vi "Start AsyncSum.vi"(7 "Opeation":string, 8 "error in (no error)":errorcluster, 9 "B":i32, 10 "A":i32, 11 "Skeleton in":refnum<class "Skeleton.lvclass">) -> (0 "error out":errorcluster, 2 "AsyncSum Event Register":refnum<event-registration>, 3 "Skeleton out":refnum<class "Skeleton.lvclass">)   [LabVIEW 2016, in "Skeleton.lvlib" / "Skeleton.lvclass"]
uses:
  Skeleton.lvclass
  Skeleton.lvclass/Skeleton.ctl
  Active Thread Configuration.ctl
  DemoSkeleton/DemoSkeleton.lvlib
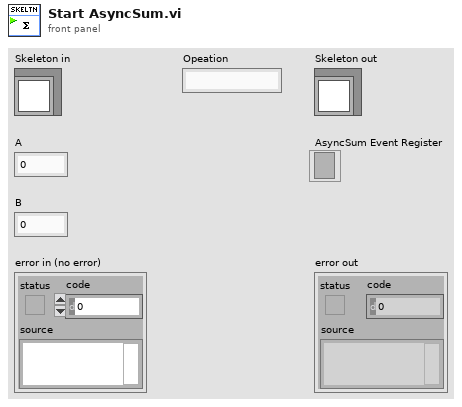
[diagram p1: front panel]
types:
  T1 = typedef "Skeleton.lvlib/Skeleton.lvclass/Active Thread Configuration.ctl" = cluster{"Operation":string, "Handle":u64, "LVUserEvent CallBack Reference":refnum<user-event>}
  T2 = typedef "Skeleton.lvlib/Skeleton.lvclass/Private Data.ctl" = cluster{"DLL path":path, "Active Thread Map":variant}
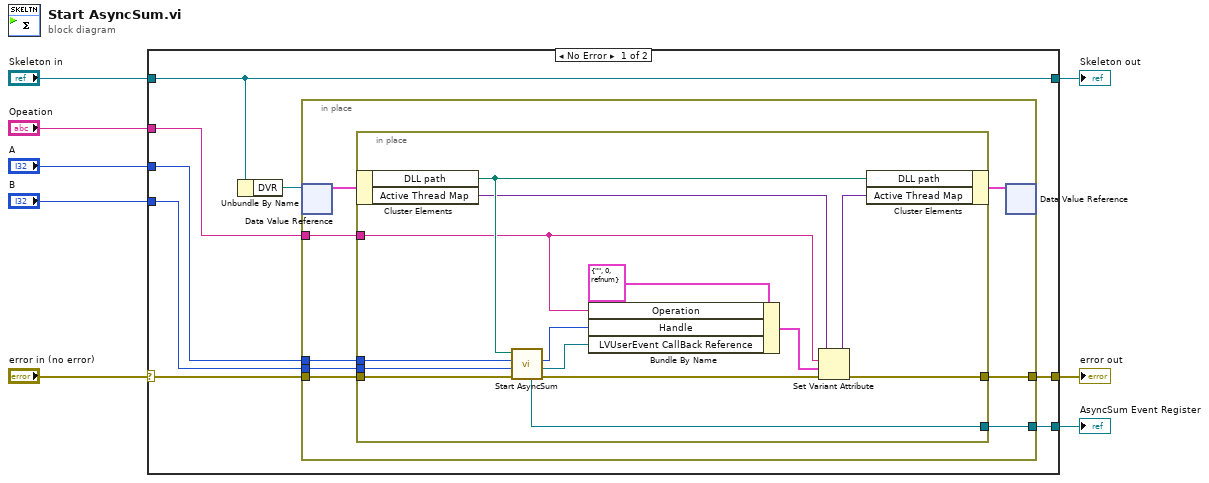
[diagram p0: block diagram]
diagram:
  n1 = case shown="No Error" "error in (no error)" {
    selector: "error in (no error)" -> [w16 w40]
    tunnel: [w15 w40] -> w8
    tunnel: [w12 w39] -> w7
    tunnel: "Skeleton in" -> [w12 w39]
    tunnel: "A" -> [w13 _]
    tunnel: "B" -> [w14 _]
    tunnel: "Opeation" -> [w10 _]
    tunnel: [w9 _] -> w1
    frame No Error {
      n2 = Unbundle By Name(w12) -> ("DVR"=w11:refnum<data-value>)
      n3 = in-place {
        in-place-border: w16 -> [w24]
        in-place-border: [w23] -> w15
        in-place-border: w14 -> [w22]
        in-place-border: w13 -> [w21]
        in-place-border: w10 -> [w18]
        in-place-border: [w17] -> w9
        n4 = in-place-dvr #1(w11) -> (w20:T2)  [unwired: 1 out]
        n5 = in-place {
          in-place-border: w24 -> [w38]
          in-place-border: [w30] -> w23
          in-place-border: w22 -> [w37]
          in-place-border: w21 -> [w36]
          in-place-border: w18 -> [w27]
          in-place-border: [w25] -> w17
          n6 = in-place-cluster #2(w20) -> ("DLL path"=w35:path, "Active Thread Map"=w29:variant)
          n7 = call "Start AsyncSum.vi"("error in (no error)"=w38, "B"=w37, "A"=w36, "path in"=w35) -> ("error out"=w31:errorcluster, "LVUserEvent CallBack Reference"=w32:refnum<user-event>, "Handle"=w33:u64, "AsyncSum Event Register"=w25:refnum<event-registration>)  [unwired: 3 in, 1 out]
          n8 = Bundle By Name(cluster=T1 {"Operation"="", "Handle"=0, "LVUserEvent CallBack Reference"=refnum} ("Active Thread Configuration"), "Operation"=w27, "Handle"=w33, "LVUserEvent CallBack Reference"=w32) -> (w26:T1)
          n9 = Set Variant Attribute(Variant=w29, name=w27, value=w26, error in=w31) -> (Variant out=w28:variant, error out=w30:errorcluster)  [unwired: 1 out]
          n10 = in-place-cluster #2("DLL path"=w35, "Active Thread Map"=w28) -> (w19:T2)
        }
        n11 = in-place-dvr #1(w19) -> ()  [unwired: 2 out]
      }
    }
    frame Error {
    }
  }
  "error out" <- w8
  "Skeleton out" <- w7
  "AsyncSum Event Register" <- w1
